vi "可能的移动.vi"(1 "Y":u8, 2 "X":u8, 3 "游戏":T1) -> (0 "输出数组":bool[][](array[boolean]))   [LabVIEW 2017]
panel:
  in  "开关":bool
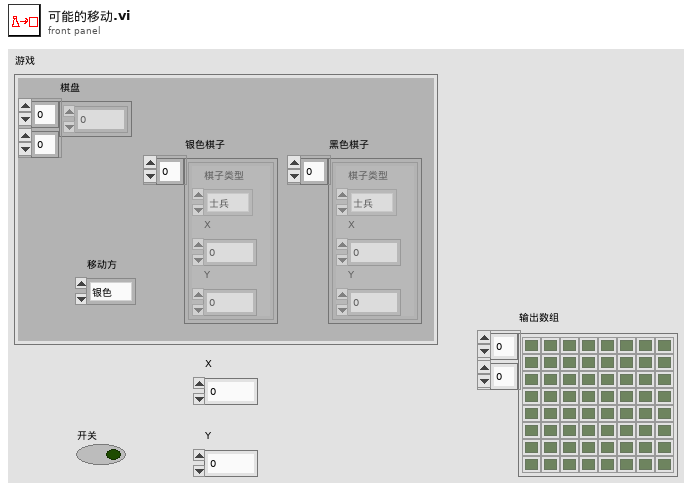
[diagram p1: front panel]
types:
  T1 = cluster{"棋盘":u16[][], "银色棋子":cluster{"棋子类型":enum16{"士兵", "骑士", "主教", "战车", "皇后", "国王", "空"}, "X":u8, "Y":u8}[], "黑色棋子":cluster{"棋子类型":enum16{"士兵", "骑士", "主教", "战车", "皇后", "国王", "空"}, "X":u8, "Y":u8}[], "移动方":enum16{"银色", "黑色"}}
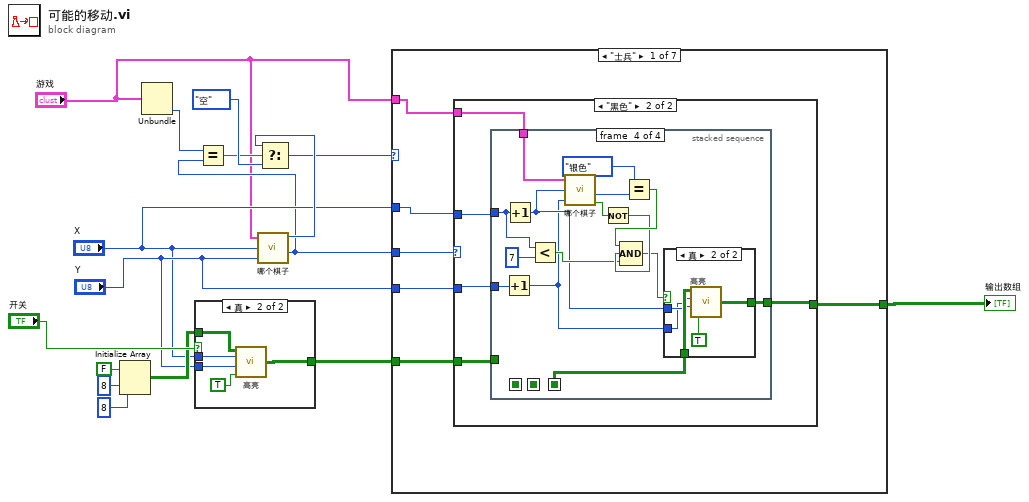
[diagram p0: block diagram]
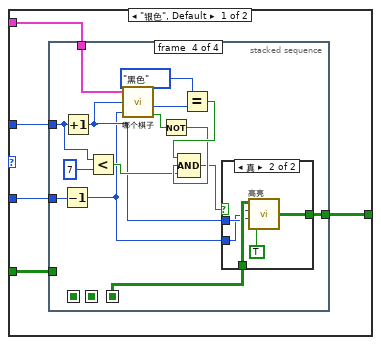
[diagram p2: hidden frame]
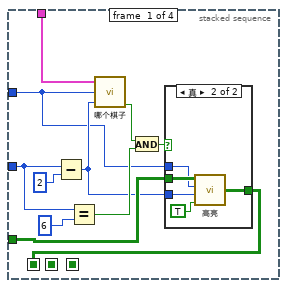
[diagram p3: hidden frame]
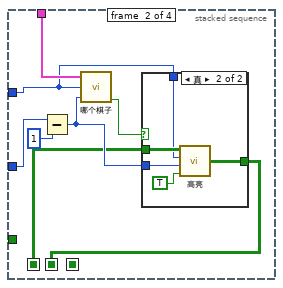
[diagram p5: hidden frame]
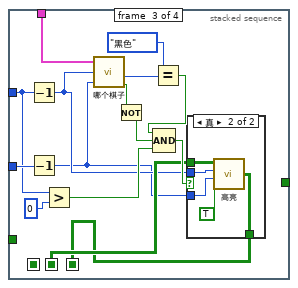
[diagram p7: hidden frame]
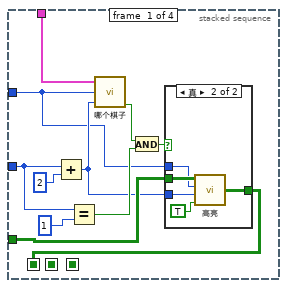
[diagram p10: hidden frame]
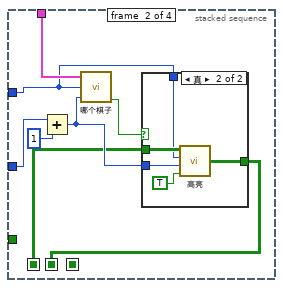
[diagram p12: hidden frame]
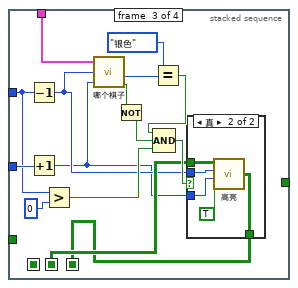
[diagram p14: hidden frame]
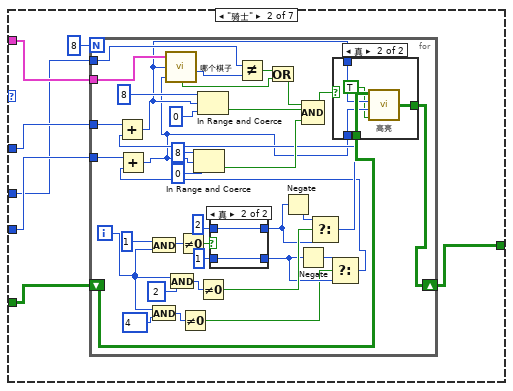
[diagram p17: hidden frame]
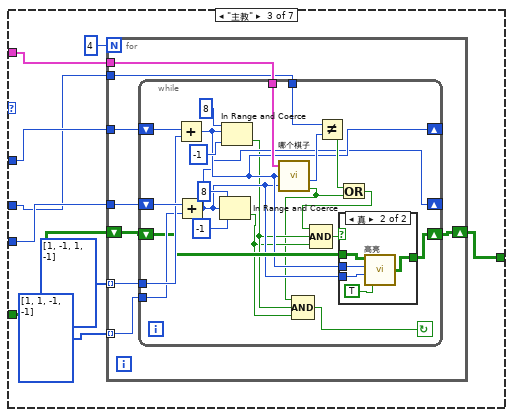
[diagram p20: hidden frame]
diagram:
  n1 = Initialize Array(FALSE, 8 ("维数大小"), 8 ("维数大小")) -> (w8:bool[][])
  n2 = Unbundle("游戏") -> ("移动方"=w16:enum16{"银色", "黑色"})  [unwired: 3 out]
  n3 = case shown="真" "开关" {
    tunnel: w8 -> [w17 w22]
    tunnel: "Y" -> [_ w20]
    tunnel: "X" -> [_ w19]
    tunnel: [w17 w18] -> w3
    frame False {
    }
    frame True {
      n4 = call "高亮.vi"("使能"=TRUE, "Y"=w20, "X"=w19, "进入的数组"=w22) -> ("输出数组"=w18:bool[][])
    }
  }
  n5 = call "哪个棋子.vi"("游戏"="游戏", "X"="X", "Y"="Y") -> ("棋子类型"=w15:enum16{"士兵", "骑士", "主教", "战车", "皇后", "国王", "空"}, "棋子颜色"=w4:enum16{"银色", "黑色"})  [unwired: 2 out]
  n6 = Equal?(x=w16, y=w4) -> (x = y?=w13:bool)
  n7 = Select(t=w15, s=w13, f=enum16{"士兵", "骑士", "主教", "战车", "皇后", "国王", "空"}."空") -> (s? t:f=w7:enum16{"士兵", "骑士", "主教", "战车", "皇后", "国王", "空"})
  n8 = case shown="\"士兵\"" w7 {
    tunnel: "Y" -> [w25 w187 w245 w286 w331 w377 _]
    tunnel: "X" -> [w26 w188 w246 w287 w333 w379 _]
    tunnel: w4 -> [w28 w186 w241 w285 w332 w378 _]
    tunnel: w3 -> [w24 w190 w240 w284 w330 w376 w410]
    tunnel: "游戏" -> [w27 w189 w242 w288 w334 w380 _]
    tunnel: [w23 w185 w239 w289 w329 w374 w410] -> w1
    frame "士兵" {
      n9 = case shown="\"黑色\"" w28 {
        tunnel: w27 -> [w33 w111]
        tunnel: w26 -> [w32 w110]
        tunnel: w25 -> [w31 w109]
        tunnel: w24 -> [w30 w108]
        tunnel: [w29 w107] -> w23
        frame "银色", Default {
          n10 = stacked-sequence {
            seq-local: [w34 _ _ _] -> [_ w52 _ _]
            seq-local: [_ w51 _ _] -> [_ _ w68 _]
            seq-local: [_ _ w65 _] -> [_ _ _ w89]
            tunnel: w33 -> [w44 w58 w79 w100]
            tunnel: w32 -> [w35 w54 w72 w93]
            tunnel: w31 -> [w41 w57 w78 w99]
            tunnel: w30 -> [w37 _ _ _]
            tunnel: [_ _ _ w86] -> w29
            frame #0 {
              n11 = Subtract(x=w41, y=u8 2) -> (x-y=w36:u8)
              n12 = Equal?(x=w41, y=u8 6) -> (x = y?=w39:bool)
              n13 = call "哪个棋子.vi"("游戏"=w44, "X"=w35, "Y"=w36) -> ("是否为空"=w42:bool)  [unwired: 3 out]
              n14 = And(x=w42, y=w39) -> (x .and. y?=w38:bool)
              n15 = case shown="真" w38 {
                tunnel: w37 -> [w45 w50]
                tunnel: w36 -> [_ w49]
                tunnel: w35 -> [_ w48]
                tunnel: [w45 w46] -> w34
                frame False {
                }
                frame True {
                  n16 = call "高亮.vi"("使能"=TRUE, "Y"=w49, "X"=w48, "进入的数组"=w50) -> ("输出数组"=w46:bool[][])
                }
              }
            }
            frame #1 {
              n17 = Subtract(x=w57, y=u8 1) -> (x-y=w53:u8)
              n18 = call "哪个棋子.vi"("游戏"=w58, "X"=w54, "Y"=w53) -> ("是否为空"=w55:bool)  [unwired: 3 out]
              n19 = case shown="真" w55 {
                tunnel: w52 -> [w59 w64]
                tunnel: w54 -> [_ w63]
                tunnel: w53 -> [_ w62]
                tunnel: [w59 w60] -> w51
                frame False {
                }
                frame True {
                  n20 = call "高亮.vi"("使能"=TRUE, "Y"=w62, "X"=w63, "进入的数组"=w64) -> ("输出数组"=w60:bool[][])
                }
              }
            }
            frame #2 {
              n21 = Decrement(x=w72) -> (x-1=w67:u8)
              n22 = Decrement(x=w78) -> (x-1=w66:u8)
              n23 = Greater?(x=w72, y=u8 0) -> (0:w70:bool)
              n24 = call "哪个棋子.vi"("游戏"=w79, "X"=w67, "Y"=w66) -> ("棋子颜色"=w77:enum16{"银色", "黑色"}, "是否为空"=w75:bool)  [unwired: 2 out]
              n25 = Not(x=w75) -> (.not. x?=w73:bool)
              n26 = Equal?(x=enum16{"银色", "黑色"}."黑色", y=w77) -> (x = y?=w74:bool)
              n27 = Compound Arithmetic op=AND ("复合运算")(w74, w73, w70) -> (w69:bool)
              n28 = case shown="真" w69 {
                tunnel: w68 -> [w80 w85]
                tunnel: w67 -> [_ w84]
                tunnel: w66 -> [_ w83]
                tunnel: [w80 w81] -> w65
                frame False {
                }
                frame True {
                  n29 = call "高亮.vi"("使能"=TRUE, "Y"=w83, "X"=w84, "进入的数组"=w85) -> ("输出数组"=w81:bool[][])
                }
              }
            }
            frame #3 {
              n30 = Decrement(x=w99) -> (x-1=w87:u8)
              n31 = Increment(x=w93) -> (x+1=w88:u8)
              n32 = Less?(x=w93, y=u8 7) -> (x < y?=w91:bool)
              n33 = call "哪个棋子.vi"("游戏"=w100, "X"=w88, "Y"=w87) -> ("棋子颜色"=w98:enum16{"银色", "黑色"}, "是否为空"=w96:bool)  [unwired: 2 out]
              n34 = Not(x=w96) -> (.not. x?=w94:bool)
              n35 = Equal?(x=enum16{"银色", "黑色"}."黑色", y=w98) -> (x = y?=w95:bool)
              n36 = Compound Arithmetic op=AND ("复合运算")(w95, w94, w91) -> (w90:bool)
              n37 = case shown="真" w90 {
                tunnel: w89 -> [w101 w106]
                tunnel: w88 -> [_ w105]
                tunnel: w87 -> [_ w104]
                tunnel: [w101 w102] -> w86
                frame False {
                }
                frame True {
                  n38 = call "高亮.vi"("使能"=TRUE, "Y"=w104, "X"=w105, "进入的数组"=w106) -> ("输出数组"=w102:bool[][])
                }
              }
            }
          }
        }
        frame "黑色" {
          n39 = stacked-sequence {
            seq-local: [w112 _ _ _] -> [_ w130 _ _]
            seq-local: [_ w129 _ _] -> [_ _ w146 _]
            seq-local: [_ _ w143 _] -> [_ _ _ w167]
            tunnel: w111 -> [w122 w136 w157 w178]
            tunnel: w110 -> [w113 w132 w150 w171]
            tunnel: w109 -> [w119 w135 w156 w177]
            tunnel: w108 -> [w115 _ _ _]
            tunnel: [_ _ _ w164] -> w107
            frame #0 {
              n40 = Add(x=w119, y=u8 2) -> (x+y=w114:u8)
              n41 = Equal?(x=w119, y=u8 1) -> (x = y?=w117:bool)
              n42 = call "哪个棋子.vi"("游戏"=w122, "X"=w113, "Y"=w114) -> ("是否为空"=w120:bool)  [unwired: 3 out]
              n43 = And(x=w120, y=w117) -> (x .and. y?=w116:bool)
              n44 = case shown="真" w116 {
                tunnel: w115 -> [w123 w128]
                tunnel: w114 -> [_ w127]
                tunnel: w113 -> [_ w126]
                tunnel: [w123 w124] -> w112
                frame False {
                }
                frame True {
                  n45 = call "高亮.vi"("使能"=TRUE, "Y"=w127, "X"=w126, "进入的数组"=w128) -> ("输出数组"=w124:bool[][])
                }
              }
            }
            frame #1 {
              n46 = Add(x=w135, y=u8 1) -> (x+y=w131:u8)
              n47 = call "哪个棋子.vi"("游戏"=w136, "X"=w132, "Y"=w131) -> ("是否为空"=w133:bool)  [unwired: 3 out]
              n48 = case shown="真" w133 {
                tunnel: w130 -> [w137 w142]
                tunnel: w132 -> [_ w141]
                tunnel: w131 -> [_ w140]
                tunnel: [w137 w138] -> w129
                frame False {
                }
                frame True {
                  n49 = call "高亮.vi"("使能"=TRUE, "Y"=w140, "X"=w141, "进入的数组"=w142) -> ("输出数组"=w138:bool[][])
                }
              }
            }
            frame #2 {
              n50 = Decrement(x=w150) -> (x-1=w145:u8)
              n51 = Increment(x=w156) -> (x+1=w144:u8)
              n52 = Greater?(x=w150, y=u8 0) -> (0:w148:bool)
              n53 = call "哪个棋子.vi"("游戏"=w157, "X"=w145, "Y"=w144) -> ("棋子颜色"=w155:enum16{"银色", "黑色"}, "是否为空"=w153:bool)  [unwired: 2 out]
              n54 = Not(x=w153) -> (.not. x?=w151:bool)
              n55 = Equal?(x=enum16{"银色", "黑色"}."银色", y=w155) -> (x = y?=w152:bool)
              n56 = Compound Arithmetic op=AND ("复合运算")(w152, w151, w148) -> (w147:bool)
              n57 = case shown="真" w147 {
                tunnel: w146 -> [w158 w163]
                tunnel: w145 -> [_ w162]
                tunnel: w144 -> [_ w161]
                tunnel: [w158 w159] -> w143
                frame False {
                }
                frame True {
                  n58 = call "高亮.vi"("使能"=TRUE, "Y"=w161, "X"=w162, "进入的数组"=w163) -> ("输出数组"=w159:bool[][])
                }
              }
            }
            frame #3 {
              n59 = Increment(x=w177) -> (x+1=w165:u8)
              n60 = Increment(x=w171) -> (x+1=w166:u8)
              n61 = Less?(x=w171, y=u8 7) -> (x < y?=w169:bool)
              n62 = call "哪个棋子.vi"("游戏"=w178, "X"=w166, "Y"=w165) -> ("棋子颜色"=w176:enum16{"银色", "黑色"}, "是否为空"=w174:bool)  [unwired: 2 out]
              n63 = Not(x=w174) -> (.not. x?=w172:bool)
              n64 = Equal?(x=enum16{"银色", "黑色"}."银色", y=w176) -> (x = y?=w173:bool)
              n65 = Compound Arithmetic op=AND ("复合运算")(w173, w172, w169) -> (w168:bool)
              n66 = case shown="真" w168 {
                tunnel: w167 -> [w179 w184]
                tunnel: w166 -> [_ w183]
                tunnel: w165 -> [_ w182]
                tunnel: [w179 w180] -> w164
                frame False {
                }
                frame True {
                  n67 = call "高亮.vi"("使能"=TRUE, "Y"=w182, "X"=w183, "进入的数组"=w184) -> ("输出数组"=w180:bool[][])
                }
              }
            }
          }
        }
      }
    }
    frame "骑士" {
      n68 = for {
        N: 8 -> [_]
        shift-right: [w212] -> w185
        shift-left: w190 -> [w213]
        tunnel: w189 -> [w228]
        tunnel: w188 -> [w227]
        tunnel: w187 -> [w226]
        tunnel: w186 -> [w221]
        i -> [w196]
        n69 = And(x=1, y=w196) -> (x .and. y?=w209:i32)
        n70 = And(x=w196, y=4 ("x")) -> (x .and. y?=w203:i32)
        n71 = And(x=w196, y=2 ("x")) -> (x .and. y?=w204:i32)
        n72 = Not Equal To 0?(x=w209) -> (x != 0?=w210:bool)
        n73 = Not Equal To 0?(x=w203) -> (x != 0?=w199:bool)
        n74 = Not Equal To 0?(x=w204) -> (x != 0?=w202:bool)
        n75 = case shown="真" w210 {
          tunnel: 1 -> [w229 w231]
          tunnel: 2 -> [w230 w232]
          tunnel: [w229 w232] -> w194
          tunnel: [w230 w231] -> w201
          frame False {
          }
          frame True {
          }
        }
        n76 = Negate(x=w194) -> (-x=w195:i32)
        n77 = Negate(x=w201) -> (-x=w200:i32)
        n78 = Select(t=w195, s=w202, f=w194) -> (s? t:f=w198:i32)
        n79 = Add(x=w227, y=w198) -> (x+y=w193:i32)
        n80 = In Range and Coerce(upper limit=8 ("上限"), x=w193, lower limit=0 ("下限")) -> (In Range?=w216:bool)  [unwired: 1 out]
        n81 = Select(t=w200, s=w199, f=w201) -> (s? t:f=w197:i32)
        n82 = Add(x=w226, y=w197) -> (x+y=w192:i32)
        n83 = call "哪个棋子.vi"("游戏"=w228, "X"=w193, "Y"=w192) -> ("棋子颜色"=w220:enum16{"银色", "黑色"}, "是否为空"=w219:bool)  [unwired: 2 out]
        n84 = In Range and Coerce(upper limit=8 ("上限"), x=w192, lower limit=0 ("下限")) -> (In Range?=w215:bool)  [unwired: 1 out]
        n85 = Not Equal?(x=w221, y=w220) -> (x != y?=w218:bool)
        n86 = Or(x=w218, y=w219) -> (x .or. y?=w217:bool)
        n87 = Compound Arithmetic op=AND ("复合运算")(w217, w216, w215) -> (w214:bool)
        n88 = case shown="真" w214 {
          tunnel: w213 -> [w233 w238]
          tunnel: w193 -> [_ w237]
          tunnel: w192 -> [_ w236]
          tunnel: [w233 w234] -> w212
          frame False {
          }
          frame True {
            n89 = call "高亮.vi"("使能"=TRUE, "Y"=w236, "X"=w237, "进入的数组"=w238) -> ("输出数组"=w234:bool[][])
          }
        }
      }
    }
    frame "主教" {
      n90 = for {
        N: 4 -> [_]
        tunnel: w246 -> [w255]
        tunnel: w245 -> [w254]
        tunnel: i32[] [1, -1, 1, -1] -> [w253] mode=indexing
        tunnel: i32[] [1, 1, -1, -1] -> [w252] mode=indexing
        tunnel: w242 -> [w251]
        tunnel: w241 -> [w250]
        shift-right: [w248] -> w239
        shift-left: w240 -> [w249]
        n91 = while {
          shift-right: [w261] -> _
          shift-left: w255 -> [w277]
          shift-right: [w260] -> _
          shift-left: w254 -> [w276]
          tunnel: w253 -> [w275]
          tunnel: w252 -> [w274]
          tunnel: w251 -> [w269]
          tunnel: w250 -> [w267]
          shift-right: [w262] -> w248
          shift-left: w249 -> [w263]
          stop <- w256 continue-if-true
          n92 = Add(x=w277, y=w275) -> (x+y=w261:i32)
          n93 = Add(x=w276, y=w274) -> (x+y=w260:i32)
          n94 = In Range and Coerce(upper limit=8 ("上限"), x=w260, lower limit=-1 ("下限")) -> (In Range?=w258:bool)  [unwired: 1 out]
          n95 = In Range and Coerce(upper limit=8 ("上限"), x=w261, lower limit=-1 ("下限")) -> (In Range?=w259:bool)  [unwired: 1 out]
          n96 = call "哪个棋子.vi"("游戏"=w269, "X"=w261, "Y"=w260) -> ("棋子颜色"=w268:enum16{"银色", "黑色"}, "是否为空"=w257:bool)  [unwired: 2 out]
          n97 = Compound Arithmetic op=AND ("复合运算")(w257, w259, w258) -> (w256:bool)
          n98 = Not Equal?(x=w267, y=w268) -> (x != y?=w266:bool)
          n99 = Or(x=w266, y=w257) -> (x .or. y?=w265:bool)
          n100 = Compound Arithmetic op=AND ("复合运算")(w265, w259, w258) -> (w264:bool)
          n101 = case shown="真" w264 {
            tunnel: w263 -> [w278 w283]
            tunnel: [w278 w282] -> w262
            tunnel: w261 -> [_ w281]
            tunnel: w260 -> [_ w280]
            frame False {
            }
            frame True {
              n102 = call "高亮.vi"("使能"=TRUE, "Y"=w280, "X"=w281, "进入的数组"=w283) -> ("输出数组"=w282:bool[][])
            }
          }
        }
      }
    }
    frame "战车" {
      n103 = for {
        N: 4 -> [_]
        tunnel: w287 -> [w300]
        tunnel: w286 -> [w299]
        tunnel: i32[] [1, 0, -1, 0] -> [w298] mode=indexing
        tunnel: i32[] [0, 1, 0, -1] -> [w297] mode=indexing
        tunnel: w288 -> [w296]
        tunnel: w285 -> [w295]
        shift-right: [w293] -> w289
        shift-left: w284 -> [w294]
        n104 = while {
          shift-right: [w306] -> _
          shift-left: w300 -> [w322]
          shift-right: [w305] -> _
          shift-left: w299 -> [w321]
          tunnel: w298 -> [w320]
          tunnel: w297 -> [w319]
          tunnel: w296 -> [w314]
          tunnel: w295 -> [w312]
          shift-right: [w307] -> w293
          shift-left: w294 -> [w308]
          stop <- w301 continue-if-true
          n105 = Add(x=w322, y=w320) -> (x+y=w306:i32)
          n106 = Add(x=w321, y=w319) -> (x+y=w305:i32)
          n107 = In Range and Coerce(upper limit=8 ("上限"), x=w305, lower limit=-1 ("下限")) -> (In Range?=w303:bool)  [unwired: 1 out]
          n108 = In Range and Coerce(upper limit=8 ("上限"), x=w306, lower limit=-1 ("下限")) -> (In Range?=w304:bool)  [unwired: 1 out]
          n109 = call "哪个棋子.vi"("游戏"=w314, "X"=w306, "Y"=w305) -> ("棋子颜色"=w313:enum16{"银色", "黑色"}, "是否为空"=w302:bool)  [unwired: 2 out]
          n110 = Compound Arithmetic op=AND ("复合运算")(w302, w304, w303) -> (w301:bool)
          n111 = Not Equal?(x=w312, y=w313) -> (x != y?=w311:bool)
          n112 = Or(x=w311, y=w302) -> (x .or. y?=w310:bool)
          n113 = Compound Arithmetic op=AND ("复合运算")(w310, w304, w303) -> (w309:bool)
          n114 = case shown="真" w309 {
            tunnel: w308 -> [w323 w328]
            tunnel: [w323 w327] -> w307
            tunnel: w306 -> [_ w326]
            tunnel: w305 -> [_ w325]
            frame False {
            }
            frame True {
              n115 = call "高亮.vi"("使能"=TRUE, "Y"=w325, "X"=w326, "进入的数组"=w328) -> ("输出数组"=w327:bool[][])
            }
          }
        }
      }
    }
    frame "皇后" {
      n116 = for {
        N: 8 -> [_]
        tunnel: w333 -> [w345]
        tunnel: w331 -> [w344]
        tunnel: i32[] [1, 0, -1, 0, -1, 1, -1, 1] -> [w343] mode=indexing
        tunnel: i32[] [0, 1, 0, -1, -1, -1, 1, 1] -> [w342] mode=indexing
        tunnel: w334 -> [w341]
        tunnel: w332 -> [w340]
        shift-right: [w338] -> w329
        shift-left: w330 -> [w339]
        n117 = while {
          shift-right: [w351] -> _
          shift-left: w345 -> [w367]
          shift-right: [w350] -> _
          shift-left: w344 -> [w366]
          tunnel: w343 -> [w365]
          tunnel: w342 -> [w364]
          tunnel: w341 -> [w359]
          tunnel: w340 -> [w357]
          shift-right: [w352] -> w338
          shift-left: w339 -> [w353]
          stop <- w346 continue-if-true
          n118 = Add(x=w367, y=w365) -> (x+y=w351:i32)
          n119 = Add(x=w366, y=w364) -> (x+y=w350:i32)
          n120 = In Range and Coerce(upper limit=8 ("上限"), x=w350, lower limit=-1 ("下限")) -> (In Range?=w348:bool)  [unwired: 1 out]
          n121 = In Range and Coerce(upper limit=8 ("上限"), x=w351, lower limit=-1 ("下限")) -> (In Range?=w349:bool)  [unwired: 1 out]
          n122 = call "哪个棋子.vi"("游戏"=w359, "X"=w351, "Y"=w350) -> ("棋子颜色"=w358:enum16{"银色", "黑色"}, "是否为空"=w347:bool)  [unwired: 2 out]
          n123 = Compound Arithmetic op=AND ("复合运算")(w347, w349, w348) -> (w346:bool)
          n124 = Not Equal?(x=w357, y=w358) -> (x != y?=w356:bool)
          n125 = Or(x=w356, y=w347) -> (x .or. y?=w355:bool)
          n126 = Compound Arithmetic op=AND ("复合运算")(w355, w349, w348) -> (w354:bool)
          n127 = case shown="真" w354 {
            tunnel: w353 -> [w368 w373]
            tunnel: [w368 w372] -> w352
            tunnel: w351 -> [_ w371]
            tunnel: w350 -> [_ w370]
            frame False {
            }
            frame True {
              n128 = call "高亮.vi"("使能"=TRUE, "Y"=w370, "X"=w371, "进入的数组"=w373) -> ("输出数组"=w372:bool[][])
            }
          }
        }
      }
    }
    frame "国王" {
      n129 = for {
        N: 8 -> [_]
        tunnel: w379 -> [w403]
        tunnel: w377 -> [w402]
        tunnel: i32[] [1, 0, -1, 0, -1, 1, -1, 1] -> [w401] mode=indexing
        tunnel: i32[] [0, 1, 0, -1, -1, -1, 1, 1] -> [w400] mode=indexing
        tunnel: w380 -> [w399]
        tunnel: w378 -> [w398]
        shift-right: [w396] -> w374
        shift-left: w376 -> [w397]
        n130 = Add(x=w403, y=w401) -> (x+y=w387:i32)
        n131 = Add(x=w402, y=w400) -> (x+y=w386:i32)
        n132 = In Range and Coerce(upper limit=7 ("上限"), x=w386, lower limit=0 ("下限")) -> (In Range?=w384:bool)  [unwired: 1 out]
        n133 = In Range and Coerce(upper limit=7 ("上限"), x=w387, lower limit=0 ("下限")) -> (In Range?=w385:bool)  [unwired: 1 out]
        n134 = call "哪个棋子.vi"("游戏"=w399, "X"=w387, "Y"=w386) -> ("棋子颜色"=w391:enum16{"银色", "黑色"}, "是否为空"=w383:bool)  [unwired: 2 out]
        n135 = Not Equal?(x=w398, y=w391) -> (x != y?=w390:bool)
        n136 = Or(x=w390, y=w383) -> (x .or. y?=w389:bool)
        n137 = Compound Arithmetic op=AND ("复合运算")(w389, w385, w384) -> (w388:bool)
        n138 = case shown="真" w388 {
          tunnel: w397 -> [w404 w409]
          tunnel: [w404 w408] -> w396
          tunnel: w387 -> [_ w407]
          tunnel: w386 -> [_ w406]
          frame False {
          }
          frame True {
            n139 = call "高亮.vi"("使能"=TRUE, "Y"=w406, "X"=w407, "进入的数组"=w409) -> ("输出数组"=w408:bool[][])
          }
        }
      }
    }
    frame "空", Default {
    }
  }
  "输出数组" <- w1
